vi "PagerTest.vi"(0 "offset":dbl=135.0, 1 "Init":bool, 2 "sample rate":dbl=48000.0, 3 "number of samples":i32=1024, 4 "Upper Cut-Off":dbl=300.0, 5 "Lower Cut-Off":dbl=150.0, 7 "error in":errorcluster) -> (13 "error out":errorcluster={"status"=FALSE, "code"=20352, "source"=" \"NI_MABase.lvlib:ma_array_Check Time Signal Continuity.vi:3520017\" when called from \"NI_MAPro.lvlib:IIR Filter for N Chan.vi:4290007\" "}, 14 "PASS/FAIL 4":bool=TRUE caption="PASS/FAIL", 15 "fundamental frequency":dbl=77.06053872402588 format="%.2p", 16 "fundamental amplitude":dbl=0.02381439174440461, 17 "fundamental dB output":dbl=102.53678986902258, 18 "THD":dbl=55.52856955444726 format="%.2p")   [LabVIEW 2014]
uses:
  <vilib>/measure/matone.llb/Harmonic Distortion Analyzer 1 Chan.vi
  <vilib>/express/express analysis/Spectral/Block/exnSpectralBlock spectral measurements peak poly.vi
  <vilib>/express/express analysis/Spectral/Block/exnSpectralBlock spectral measurements peak WFM.vi
  <vilib>/express/express analysis/Spectral/XNode/ExpressSpectralMeasurementsBlockNode.xnode
  <vilib>/measure/NI_MAPro.lvlib
panel:
  out "FFT Mask":dynamicdata(graph)=[{"t0"=timestamp(0 s since 1904-01-01), "dt"=2.3994001766382365, "Y"=array[10003 elements]}, {"t0"=timestamp(0 s since 1904-01-01), "dt"=2.3994001766382365, "Y"=array[10003 elements], "attributes"=variant("NI_ChannelName"=variant(string "Failures"))}, {"t0"=timestamp(0 s since 1904-01-01), "dt"=2.3994001766382365, "Y"=array[10003 elements], "attributes"=variant("NI_ChannelName"=variant(string "Upper Limit"))}, {"t0"=timestamp(0 s since 1904-01-01), "dt"=2.3994001766382365, "Y"=array[10003 elements], "attributes"=variant("NI_ChannelName"=variant(string "Lower Limit"))}]
  out "number of cycles \nbefore sample acquisition":i32=18
  out "Beeper Time Domain":waveform(dbl)(graph)={"t0"=timestamp(3557506913.4073706 s since 1904-01-01), "dt"=2.0833333101715314e-05, "Y"=array[20005 elements], "attributes"=variant("NI_ChannelName"=variant(string "Force (Trigger)"), "NI_OriginalChannelName"=variant(string "Force"), "NI_UnitDescription"=variant(string "Newtons"))}
  out "FFT Peak":cluster{"f0":dbl, "df":dbl, "magnitude":dbl[]}(graph)={"f0"=0.0, "df"=2.3994001766382365, "magnitude"=array[10003 elements]}
  # "Trigger at 0.8"
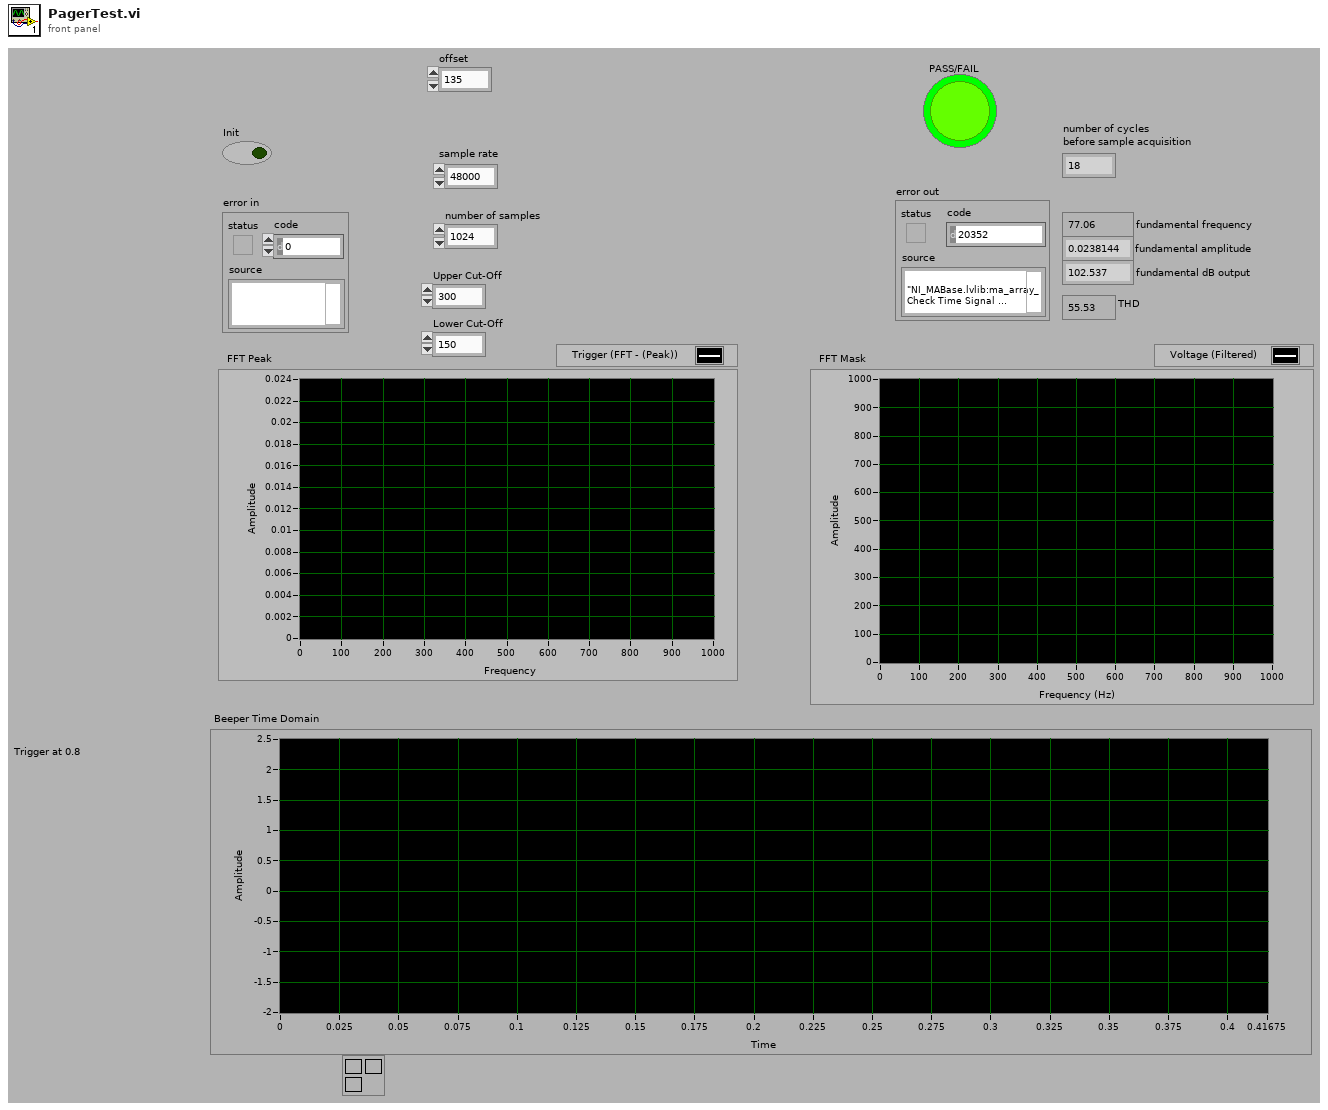
[diagram p1: front panel]
types:
  T1 = enum16{"none", "input signal", "fundamental signal", "residual signal", "harmonics only", "noise and spurs"}
  T2 = cluster{"averaging mode":u16, "weighting mode":u16, "number of averages":u32}
  T3 = cluster{"dB On (F)":bool, "unwrap phase (F)":bool, "convert to degree (F)":bool}
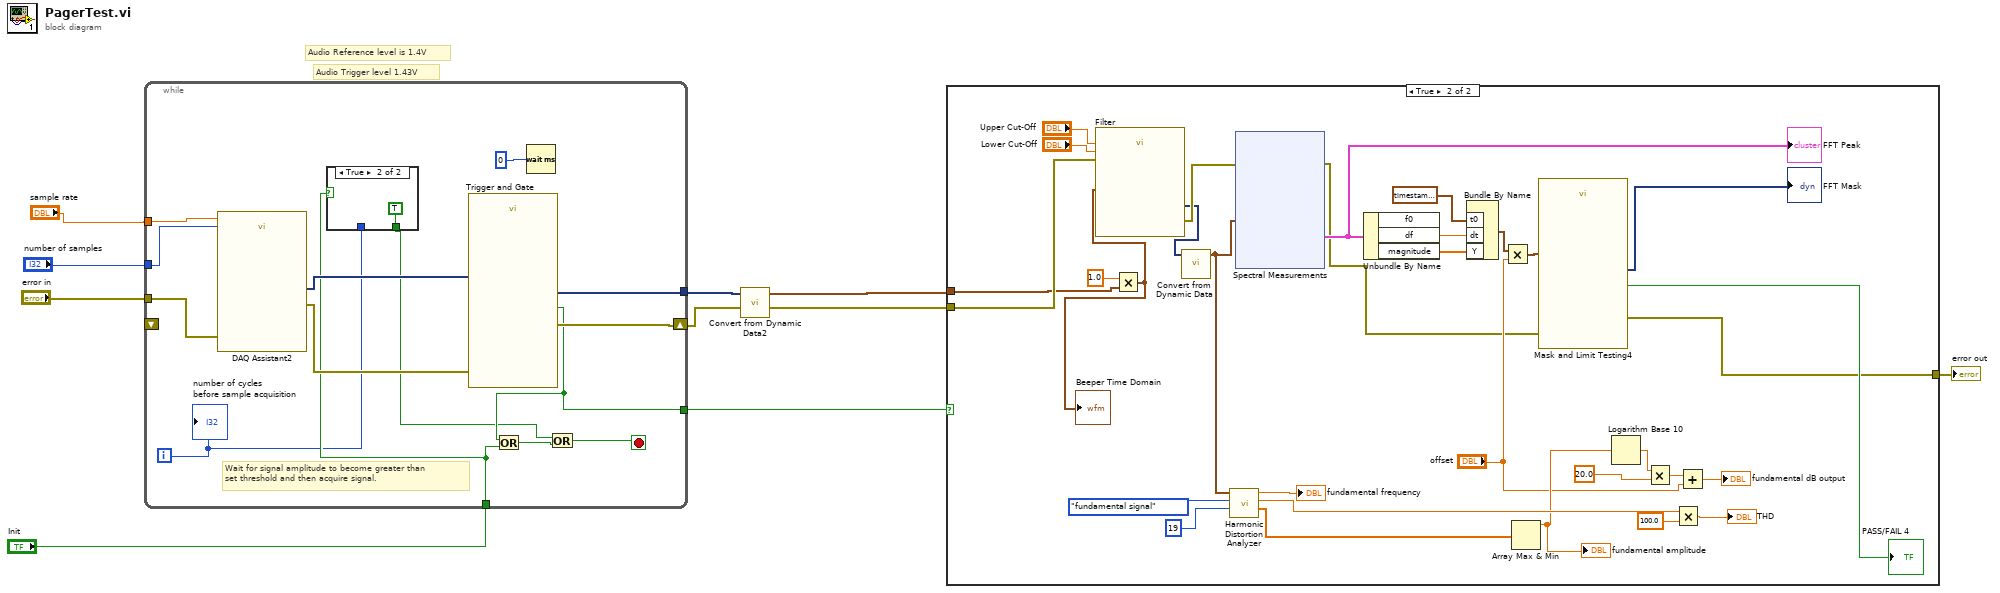
[diagram p0: block diagram]
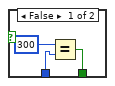
[diagram p2: hidden frame]
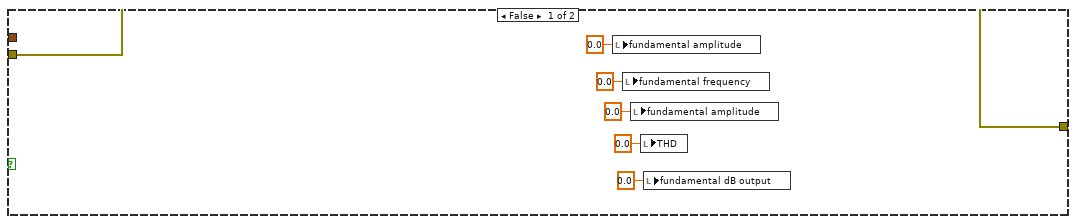
[diagram p3: hidden frame]
diagram:
  # "Audio Trigger level 1.43V"
  # "Audio Reference level is 1.4V"
  n1 = while {
    tunnel: [w15] -> w6
    shift-right: [w21] -> w5
    shift-left: _ -> [_]
    tunnel: [w23] -> w4
    tunnel: "sample rate" -> [w20]
    tunnel: "number of samples" -> [w19]
    tunnel: "error in" -> [w18]
    tunnel: "Init" -> [w14]
    i -> [w13]
    stop <- w12 stop-if-true
    # "Wait for signal amplitude to become greater than\nset threshold and then acquire signal."
    n2 = call "DAQ Assistant2"("rate"=w20, "number of samples"=w19, "error in"=w18) -> ("data"=w17:dynamicdata, "error out"=w16:errorcluster)  [unwired: 13 in, 2 out]
    n3 = case shown="True" w14 {
      tunnel: w13 -> [w26 _]
      tunnel: [w24 TRUE] -> w10
      frame False {
        n4 = Equal?(x=300, y=w26) -> (x = y?=w24:bool)
      }
      frame True {
      }
    }
    n5 = call "Trigger and Gate"("error in (no error)"=w16, "Signals"=w17) -> ("error out"=w21:errorcluster, "Triggered Signals"=w23:dynamicdata, "Data Available"=w15:bool)  [unwired: 6 in, 1 out]
    n6 = Or(x=w15, y=w14) -> (x .or. y?=w11:bool)
    n7 = Wait (ms)(milliseconds to wait=u32 0) -> ()  [unwired: 1 out]
    n8 = Or(x=w10, y=w11) -> (x .or. y?=w12:bool)
    "number of cycles \nbefore sample acquisition" <- w13
  }
  n9 = call "Convert from Dynamic Data2"("Dynamic Data Type"=w4) -> ("Waveform"=w7:waveform(dbl))  [unwired: 3 in]
  n10 = case shown="True" w6 {
    tunnel: w7 -> [_ w60]
    tunnel: w5 -> [w33 w62]
    tunnel: [w33 w63] -> w2
    frame False {
      n11 = local write "fundamental amplitude"(0.0 ("fundamental amplitude")) -> ()
      n12 = local write "fundamental frequency"(0.0 ("fundamental frequency")) -> ()
      n13 = local write "fundamental amplitude"(0.0 ("fundamental amplitude")) -> ()
      n14 = local write "THD"(0.0 ("THD")) -> ()
      n15 = local write "fundamental dB output"(0.0 ("fundamental dB output")) -> ()
    }
    frame True {
      n16 = Multiply(x=1.0, y=w60) -> (x*y=w57:waveform(dbl))
      "Beeper Time Domain" <- w57
      n17 = call "Filter"("error in (no error)"=w62, "Lower Cut-Off"="Lower Cut-Off", "Upper Cut-Off"="Upper Cut-Off", "Signal"=w57) -> ("error out"=w61:errorcluster, "Filtered Signal"=w59:dynamicdata)  [unwired: 6 in]
      n18 = call "Convert from Dynamic Data"("Dynamic Data Type"=w59) -> ("Waveform"=w38:waveform(dbl))  [unwired: 3 in]
      n19 = call-poly <vilib>:"Harmonic Distortion Analyzer.vi"("highest harmonic"=19, "export mode"=T1."fundamental signal" ("export signals"), "signal in"=w38) -> ("components level"=w50:dbl[], "THD"=w40:dbl, "detected fundamental frequency"=→"fundamental frequency":dbl)  [unwired: 3 in, 3 out]
      n20 = xnode "Spectral Measurements"("Signals"=w38, "error in (no error)"=w61) -> ("FFT - (Peak)"=w56:cluster{"f0":dbl, "df":dbl, "magnitude":dbl[]}, "error out"=w34:errorcluster)  [unwired: 1 out]
      "FFT Peak" <- w56
      n21 = Unbundle By Name(w56) -> ("df"=w55:dbl, "magnitude"=w54:dbl[])  [unwired: 1 out]
      n22 = Bundle By Name("t0"=timestamp(0 s since 1904-01-01), "dt"=w55, "Y"=w54) -> (w36:waveform(dbl))  [unwired: 1 in]
      n23 = Multiply(x=w36, y="offset") -> (x*y=w37:waveform(dbl))
      n24 = Array Max & Min(array=w50) -> (max value=w39:dbl)  [unwired: 3 out]
      "fundamental amplitude" <- w39
      n25 = call "Mask and Limit Testing4"("error in"=w34, "Signals"=w37) -> ("error out"=w63:errorcluster, "Passed"=→"PASS/FAIL 4":bool, "Tested Signals"=→"FFT Mask":dynamicdata)  [unwired: 6 in, 1 out]
      n26 = Logarithm Base 10(1:w39) -> (0:w49:dbl)
      n27 = Multiply(x=w49, y=20.0) -> (x*y=w47:dbl)
      n28 = Multiply(x=w40, y=100.0) -> (x*y=→"THD":dbl)
      n29 = Add(x=w47, y="offset") -> (x+y=→"fundamental dB output":dbl)
    }
  }
  "error out" <- w2
